vi "Configure.vi"(8 "error in (no error)":errorcluster, 11 "Analyser in":refnum<class "Analyser.lvclass">) -> (0 "error out":errorcluster, 3 "Analyser out":refnum<class "Analyser.lvclass">)   [LabVIEW 2020, in "Analyser.lvlib" / "Analyser.lvclass"]
uses:
  Analyser.lvclass
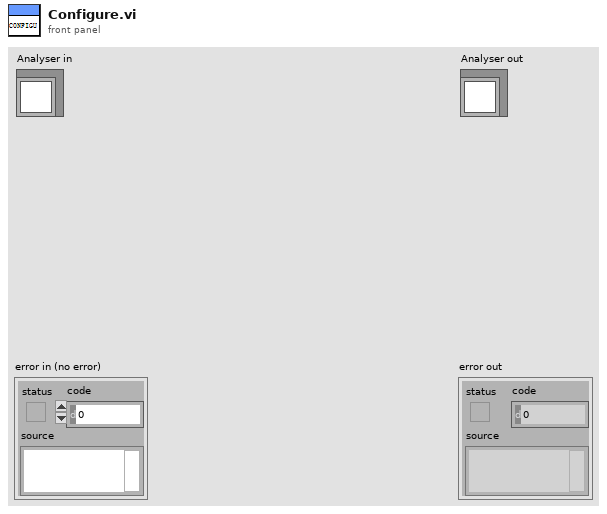
[diagram p1: front panel]
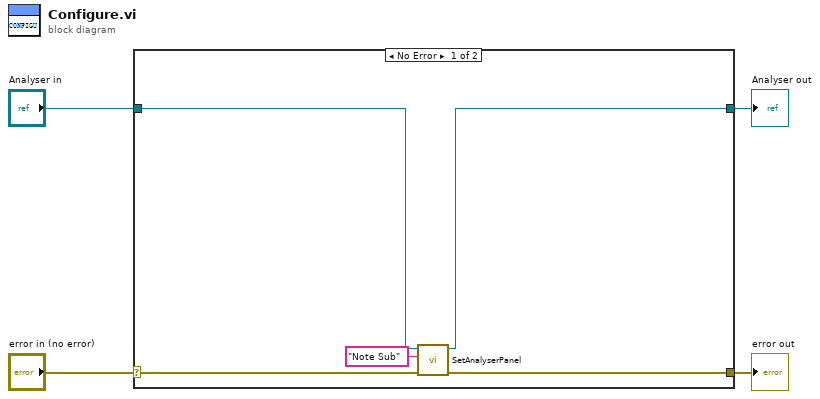
[diagram p0: block diagram]
diagram:
  n1 = case shown="No Error" "error in (no error)" {
    selector: "error in (no error)" -> [w9 w11]
    tunnel: [w8 w11] -> w3
    tunnel: [w6 w10] -> w1
    tunnel: "Analyser in" -> [w7 w10]
    frame No Error {
      n2 = call-dynamic "SetAnalyserPanel.vi"("error in (no error)"=w9, "Panel"="Note Sub", "Analyser in"=w7) -> ("error out"=w8:errorcluster, "Analyser out"=w6:refnum<class "Analyser.lvclass">)  [unwired: 7 in]
    }
    frame Error {
    }
  }
  "error out" <- w3
  "Analyser out" <- w1
